vi "S2C_UNITHERM_Proc_Initialize.vi"(7 "Local?":bool, 8 "Error In":errorcluster, 10 "Command":string, 11 "JSON String":string) -> (0 "Error Out":errorcluster, 2 "Response":variant)   [LabVIEW 2024]
uses:
  S2C_UNITHERM_Proc_Globals.vi
  <vilib>/Instr/_visa.llb/VISA Configure Serial Port (Instr).vi
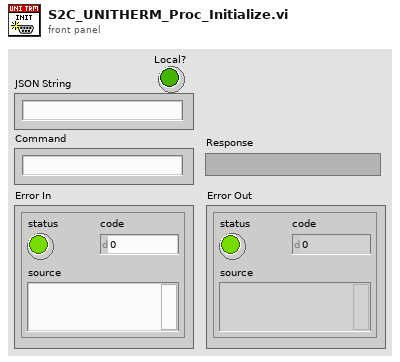
[diagram p1: front panel]
types:
  T1 = cluster{"Resource Name":string, "Baud Rate":u32, "Data Bits":u16, "Parity":u16, "Stop Bits":u16, "Flow Control":u16, "Termination Char":u8, "Enable Termination":bool, "Timeout":u32}
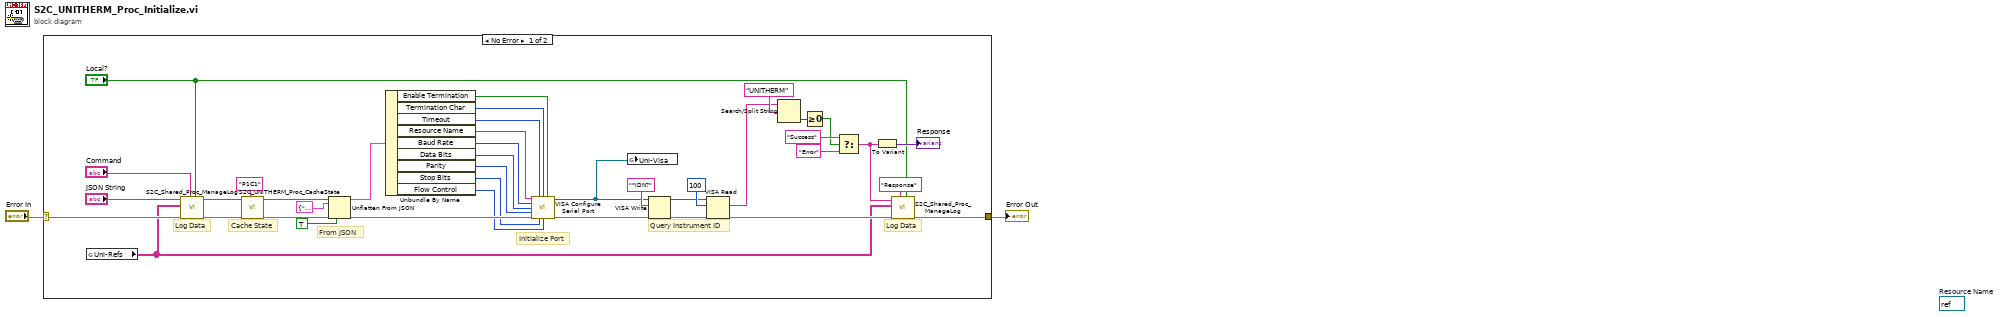
[diagram p0: block diagram]
diagram:
  (unwired) refnum<visa-resource-name> refnum  # Resource Name
  n1 = case shown="No Error" "Error In" {
    selector: "Error In" -> [w24 w43]
    tunnel: [w21 w43] -> w1
    frame No Error {
      # "Initialize Port"
      # "Cache State"
      # "Log Data"
      # "Log Data"
      # "Query Instrument ID"
      # "From JSON"
      n2 = global read "S2C_UNITHERM_Proc_Globals.vi" "Uni-Refs"() -> (w5:string[][])
      n3 = call "S2C_Shared_Proc_ManageLog.vi"("Local?"="Local?", "Command"="Command", "Error In"=w24, "Refs"=w5, "Data In"="JSON String") -> ("Error Out"=w18:errorcluster, "Data Out"=w17:string)  [unwired: 5 in]
      n4 = call "S2C_UNITHERM_Proc_CacheState.vi"("Label"="P1C1", "Error In"=w18, "Data In"=w17) -> ("Error Out"=w15:errorcluster, "Data Out"=w16:string)  [unwired: 7 in]
      n5 = Unflatten From JSON(JSON string=w16, type and defaults=T1 {"Resource Name"="", "Baud Rate"=0, "Data Bits"=5, "Parity"=0, "Stop Bits"=10, "Flow Control"=0, "Termination Char"=0, "Enable Termination"=FALSE, "Timeout"=0}, default null elements? (F)=TRUE, error in (no error)=w15) -> (value=w40:T1, error out=w30:errorcluster)  [unwired: 3 in]
      n6 = Unbundle By Name(w40) -> ("Enable Termination"=w35:bool, "Termination Char"=w36:u8, "Timeout"=w37:u32, "Resource Name"=w38:string, "Baud Rate"=w39:u32, "Data Bits"=w28:u16, "Parity"=w27:u16, "Stop Bits"=w26:u16, "Flow Control"=w25:u16)
      n7 = call-poly "VISA Configure Serial Port"("VISA resource name"=w38, "timeout (10sec)"=w37, "termination char\n(0xA = '\\n' = LF)"=w36, "Enable Termination\nChar (T)"=w35, "baud rate (9600)"=w39, "data bits (8)"=w28, "parity (0:none)"=w27, "error in (no error)"=w30, "stop bits (10: 1 bit)"=w26, "flow control (0:none)"=w25) -> ("VISA resource name out"=w4:refnum<visa-resource-name>, "error out"=w11:errorcluster)  [unwired: 4 in]
      n8 = global write "S2C_UNITHERM_Proc_Globals.vi" "Uni-Visa"(w4) -> ()
      n9 = VISA Write(VISA resource name=w4, write buffer="*IDN?", error in (no error)=w11) -> (VISA resource name out=w12:refnum<visa-resource-name>, error out=w33:errorcluster)  [unwired: 1 out]
      n10 = VISA Read(VISA resource name=w12, byte count=u32 100, error in (no error)=w33) -> (read buffer=w8:string, error out=w22:errorcluster)  [unwired: 2 out]
      n11 = Search/Split String(string=w8, search string/char (-)="UNITHERM") -> (offset of match=w9:i32)  [unwired: 1 in, 2 out]
      n12 = Greater Or Equal To 0?(x=w9) -> (x >= 0?=w7:bool)
      n13 = Select(t="Success", s=w7, f="Error") -> (s? t:f=w3:string)
      n14 = To Variant(anything=w3) -> (Variant=→"Response":variant)
      n15 = call "S2C_Shared_Proc_ManageLog.vi"("Local?"="Local?", "Command"="Response", "Error In"=w22, "Refs"=w5, "Data In"=w3) -> ("Error Out"=w21:errorcluster)  [unwired: 5 in, 1 out]
    }
    frame Error {
    }
  }
  "Error Out" <- w1
